vi "GetLaserParameters.vi"(7 "error in (no error)":errorcluster, 8 "Camera Reference in":refnum<k24>) -> (0 "FrameRangeEnd (0-100, end-start >= 25)":i32 min=0 max=100 step=1, 1 "FrameRangeStart (0-100, end-start >= 25)":i32 min=0 max=100 step=1, 2 "LaserFringeCodingMode (Fast Accurate Reflective)":u8(ring) items=["Fast", "Accurate", "Reflective"], 3 "error out":errorcluster, 5 "PowerLevel (50-100)":i32 min=0 max=100 step=1, 6 "FramePartitionCount (1-4)":i32=1 min=1 max=4 step=1)   [LabVIEW 2023]
uses:
  C:/Mech-Mind/Mech-Eye SDK-2.5.0-b5-dev-01-03/API/dll/net48/MechEyeApiNet.dll
  dll/net48/MechEyeApiNet.dll
panel:
  out "Camera Reference out":refnum<k24>
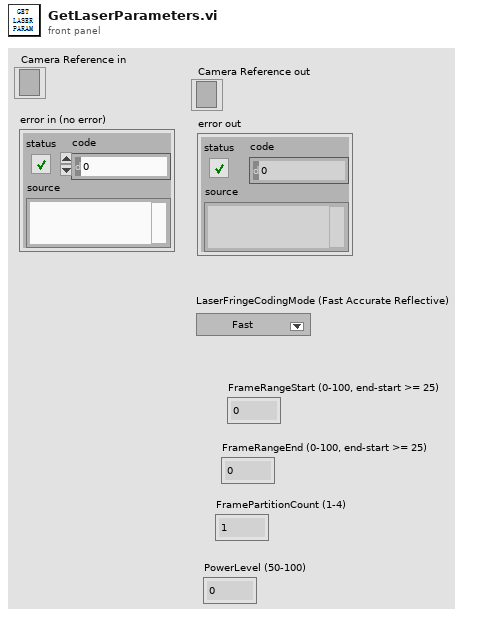
[diagram p1: front panel]
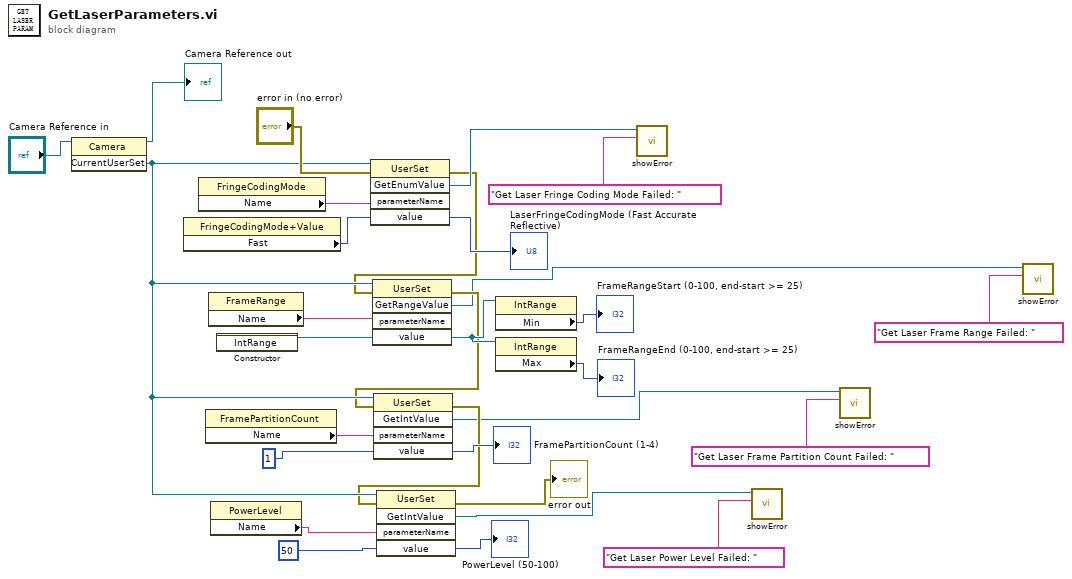
[diagram p0: block diagram]
diagram:
  n1 = invoke class="Camera" method="CurrentUserSet"(reference="Camera Reference in") -> (reference out=→"Camera Reference out":refnum<k24>, "CurrentUserSet"=w15:refnum<k24>)  [unwired: 2 in, 1 out]
  n2 = property class="FringeCodingMode+Value"() -> ("Fast"=w27:i32)  [unwired: 2 in, 2 out]
  n3 = property class="FringeCodingMode"() -> ("Name"=w28:string)  [unwired: 2 in, 2 out]
  n4 = property class="FramePartitionCount"() -> ("Name"=w17:string)  [unwired: 2 in, 2 out]
  n5 = property class="FrameRange"() -> ("Name"=w23:string)  [unwired: 2 in, 2 out]
  n6 = property class="PowerLevel"() -> ("Name"=w13:string)  [unwired: 2 in, 2 out]
  n7 = constructor class="IntRange"() -> (reference out=w22:refnum<k24>)  [unwired: 3 in, 2 out]
  n8 = invoke class="UserSet" method="GetEnumValue"(reference=w15, error in="error in (no error)", "parameterName"=w28, "value"=w27) -> (error out=w11:errorcluster, "GetEnumValue"=w26:refnum<k24>, "value"=→"LaserFringeCodingMode (Fast Accurate Reflective)":i32)  [unwired: 1 in, 2 out]
  n9 = invoke class="UserSet" method="GetRangeValue"(reference=w15, error in=w11, "parameterName"=w23, "value"=w22) -> (error out=w10:errorcluster, "GetRangeValue"=w6:refnum<k24>, "value"=w21:refnum<k24>)  [unwired: 1 in, 2 out]
  n10 = invoke class="UserSet" method="GetIntValue"(reference=w15, error in=w10, "parameterName"=w17, "value"=1) -> (error out=w9:errorcluster, "GetIntValue"=w4:refnum<k24>, "value"=→"FramePartitionCount (1-4)":i32)  [unwired: 1 in, 2 out]
  n11 = invoke class="UserSet" method="GetIntValue"(reference=w15, error in=w9, "parameterName"=w13, "value"=50) -> (error out=→"error out":errorcluster, "GetIntValue"=w2:refnum<k24>, "value"=→"PowerLevel (50-100)":i32)  [unwired: 1 in, 2 out]
  n12 = property class="IntRange"(reference=w21) -> ("Min"=→"FrameRangeStart (0-100, end-start >= 25)":i32)  [unwired: 1 in, 2 out]
  n13 = property class="IntRange"(reference=w21) -> ("Max"=→"FrameRangeEnd (0-100, end-start >= 25)":i32)  [unwired: 1 in, 2 out]
  n14 = call "showError.vi"("String"="Get Laser Fringe Coding Mode Failed: ", "MMind.Eye.ErrorStatus"=w26) -> ()  [unwired: 10 in]
  n15 = call "showError.vi"("String"="Get Laser Power Level Failed: ", "MMind.Eye.ErrorStatus"=w2) -> ()  [unwired: 10 in]
  n16 = call "showError.vi"("String"="Get Laser Frame Partition Count Failed: ", "MMind.Eye.ErrorStatus"=w4) -> ()  [unwired: 10 in]
  n17 = call "showError.vi"("String"="Get Laser Frame Range Failed: ", "MMind.Eye.ErrorStatus"=w6) -> ()  [unwired: 10 in]
